vi "ParseXMLFragments with Attributes.vi"(8 "error in (no error)":errorcluster, 9 "content":T1, 10 "XML in":string) -> (0 "error out":errorcluster, 2 "XML Elements":T2[](array[typedef]), 3 "Element Names":string[](array[string]))   [LabVIEW 2011]
doc: "This VI parses its XML code input and returns an array of the top level elements."
uses:
  Type Defs/XML Element Table - Cluster.ctl
  Type Defs/Node Info - Cluster.ctl
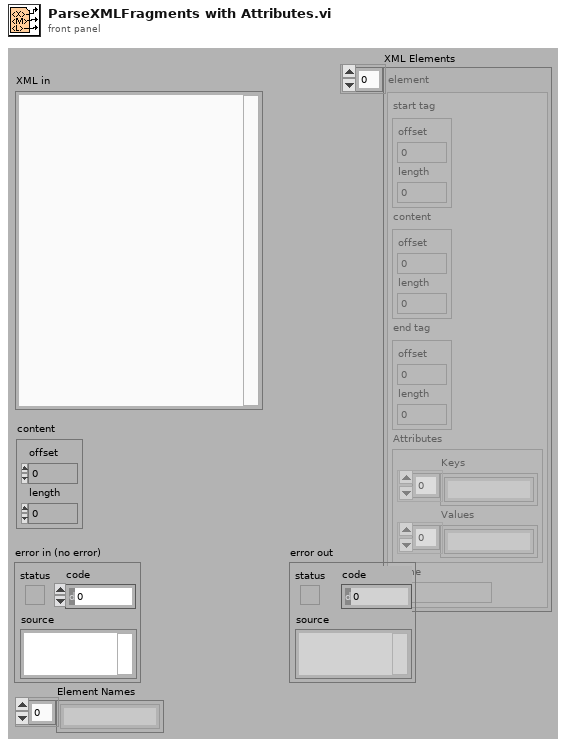
[diagram p1: front panel]
types:
  T1 = typedef "Node Info - Cluster.ctl" = cluster{"offset":i32, "length":i32}
  T2 = typedef "XML Element Table - Cluster.ctl" = cluster{"start tag":T1, "content":T1, "end tag":T1, "Attributes":cluster{"Keys":string[], "Values":string[]}, "name":string}
  T3 = cluster{"start tag":T1, "content":T1, "close tag":T1, "Attributes":cluster{"Keys":string[], "Values":string[]}, "element name":string}
  T4 = cluster{"start tag":T1, "start tag":T1, "start tag":T1, "Attributes":cluster{"Keys":string[], "Values":string[]}, "element name":string}
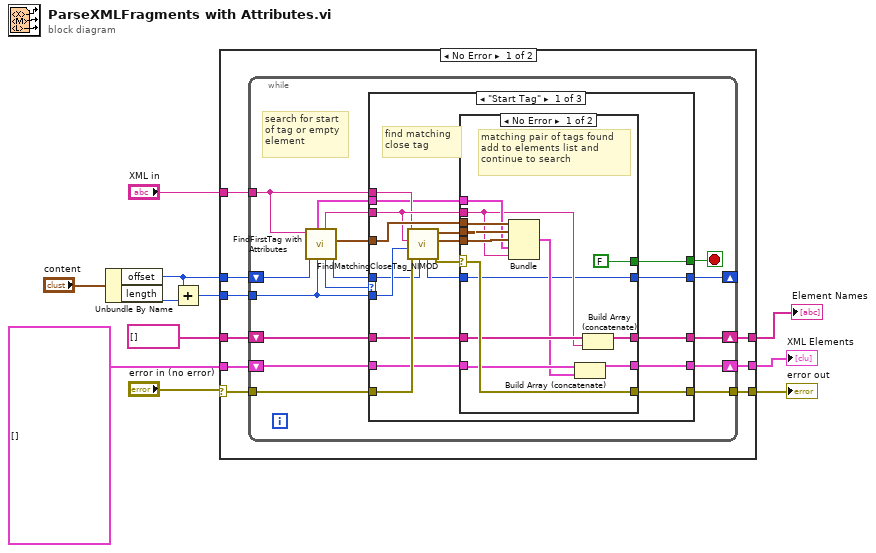
[diagram p0: block diagram]
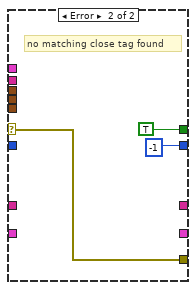
[diagram p2: hidden frame]
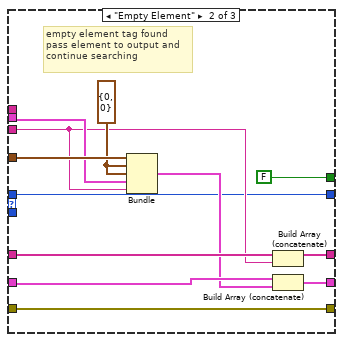
[diagram p3: hidden frame]
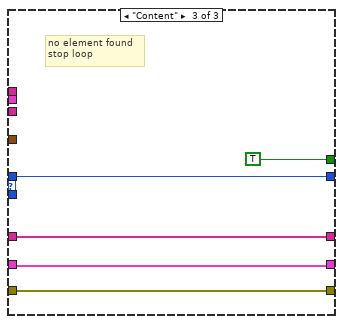
[diagram p4: hidden frame]
diagram:
  n1 = Unbundle By Name("content") -> ("offset"=w5:i32, "length"=w6:i32)
  n2 = Add(x=w5, y=w6) -> (x+y=w4:i32)
  n3 = case shown="No Error" "error in (no error)" {
    selector: "error in (no error)" -> [w18 w88]
    tunnel: "XML in" -> [w20 _]
    tunnel: string[] [] -> [w16 _]
    tunnel: [w19 _] -> w3
    tunnel: [w17 w88] -> w8
    tunnel: [w15 _] -> w1
    tunnel: w5 -> [w14 _]
    tunnel: w4 -> [w13 _]
    tunnel: T2[] [] ("XML Elements") -> [w12 _]
    frame No Error {
      n4 = while {
        shift-right: [w34] -> w19
        shift-left: w12 -> [w35]
        tunnel: w18 -> [w33]
        tunnel: [w32] -> w17
        shift-right: [w27] -> w15
        shift-left: w16 -> [w28]
        tunnel: w20 -> [w26]
        shift-right: [w22] -> _
        shift-left: w14 -> [w25]
        tunnel: w13 -> [w24]
        stop <- w36 stop-if-true
        # "search for start\nof tag or empty\nelement"
        n5 = call "FindFirstTag with Attributes.vi"("max offset"=w24, "offset (0)"=w25, "XML String In"=w26) -> ("offset past match"=w23:i32, "start tag"=w29:T1, "case"=w31:enum16{"Start Tag", "Empty Element", "Content"}, "element name"=w30:string, "Attributes"=w21:cluster{"Keys":string[], "Values":string[]})  [unwired: 4 in]
        n6 = case shown="\"Start Tag\"" w31 {
          tunnel: [w46 FALSE TRUE] -> w36
          tunnel: w35 -> [w52 w82 w85]
          tunnel: [w49 w81 w85] -> w34
          tunnel: w33 -> [w54 w80 w87]
          tunnel: [w50 w80 w87] -> w32
          tunnel: w30 -> [w44 w72 _]
          tunnel: w29 -> [w51 w76 _]
          tunnel: w28 -> [w45 w78 w84]
          tunnel: [w43 w77 w84] -> w27
          tunnel: w26 -> [w42 _ _]
          tunnel: w24 -> [w41 _ _]
          tunnel: w23 -> [w40 w71 w83]
          tunnel: [w38 w71 w83] -> w22
          tunnel: w21 -> [w37 w73 _]
          frame "Start Tag" {
            # "find matching\nclose tag"
            n7 = call "FindMatchingCloseTag_NIMOD.vi"("offset (0)"=w40, "error in"=w54, "max offset"=w41, "element name"=w44, "XML string in"=w42) -> ("error out"=w53:errorcluster, "close tag"=w47:T1, "content"=w48:T1, "offset past close tag"=w39:i32)  [unwired: 3 in]
            n8 = case shown="No Error" w53 {
              selector: w53 -> [w67 w70]
              tunnel: w48 -> [w60 _]
              tunnel: w52 -> [w66 _]
              tunnel: w51 -> [w61 _]
              tunnel: [w67 w70] -> w50
              tunnel: [w65 _] -> w49
              tunnel: w47 -> [w58 _]
              tunnel: [FALSE TRUE] -> w46
              tunnel: w45 -> [w63 _]
              tunnel: w44 -> [w56 _]
              tunnel: [w62 _] -> w43
              tunnel: w39 -> [w55 _]
              tunnel: [w55 -1 ("offset")] -> w38
              tunnel: w37 -> [w57 _]
              frame No Error {
                # "matching pair of tags found\nadd to elements list and\ncontinue to search"
                n9 = Bundle("start tag"=w61, "content"=w60, "close tag"=w58, "Attributes"=w57, "element name"=w56) -> (w59:T3)  [unwired: 1 in]
                n10 = Build Array (concatenate)(w66, w59) -> (w65:T2[])
                n11 = Build Array (concatenate)(w63, w56) -> (w62:string[])
              }
              frame Error {
                # "no matching close tag found"
              }
            }
          }
          frame "Empty Element" {
            w74 = T1 {"offset"=0, "length"=0} ("start tag")
            # "empty element tag found\npass element to output and\ncontinue searching"
            n12 = Bundle("start tag"=w76, "start tag"=w74, "start tag"=w74, "Attributes"=w73, "element name"=w72) -> (w75:T4)  [unwired: 1 in]
            n13 = Build Array (concatenate)(w78, w72) -> (w77:string[])
            n14 = Build Array (concatenate)(w82, w75) -> (w81:T2[])
          }
          frame "Content" {
            # "no element found\nstop loop"
          }
        }
      }
    }
    frame Error {
    }
  }
  "XML Elements" <- w3
  "error out" <- w8
  "Element Names" <- w1
